vi "Untitled 3.vi"() -> ()   [LabVIEW 2016]
panel:
  in  "0, 2":i16
  out "0, 1":i16
  in  "x":bool
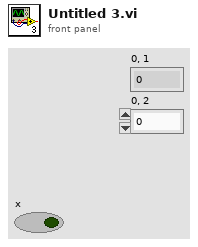
[diagram p1: front panel]
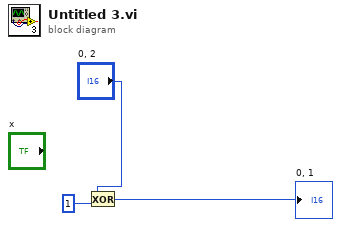
[diagram p0: block diagram]
diagram:
  n1 = Exclusive Or(1:i16 1 ("y"), 2:"0, 2") -> (0:→"0, 1":i16)
